vi "7.8-TCP Receive Server.vi"() -> ()   [LabVIEW 2010]
doc: "Sends a specified waveform through a TCP port. The VI first listens for a connection and, once established, sends the number of bytes to be sent followed by the data. After the data is sent, the VI waits for an 'all received' signal from the client and then breaks the connection.\n\n<B>Note:</B> Requires the Data Client.vi located in the same library as this VI."
uses:
  4-High Neurons/4.0-Timing Badass.ctl
  5-Forebrain/5.0-Global.vi
panel:
  out "Variant Cast":T1
  out "GUI":T1
  in  "Port":u16=53483 min=1025 step=1
  # "Instructions:\n1. Open the Data Client.vi\n2. Run This VI first.\n3. Run the Data Client.vi Second.\n4. Adjust the # of Points Function, and Noise Level controls.\n5. Observe the Chart on the Data Client.vi.\n6. Stop This VI. The Data Client.vi will time out and stop."
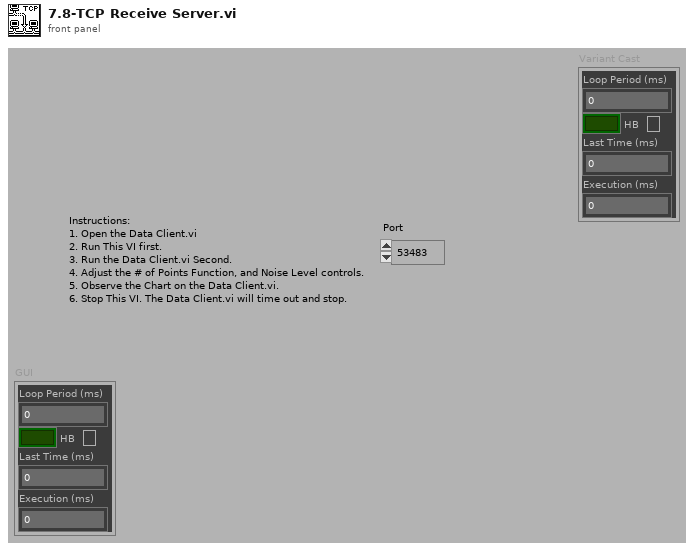
[diagram p1: front panel]
types:
  T1 = typedef "4.0-Timing Badass.ctl" = cluster{"Loop Period (ms)":u32, "HB":bool, "Last Time (ms)":u32, "Execution (ms)":u32}
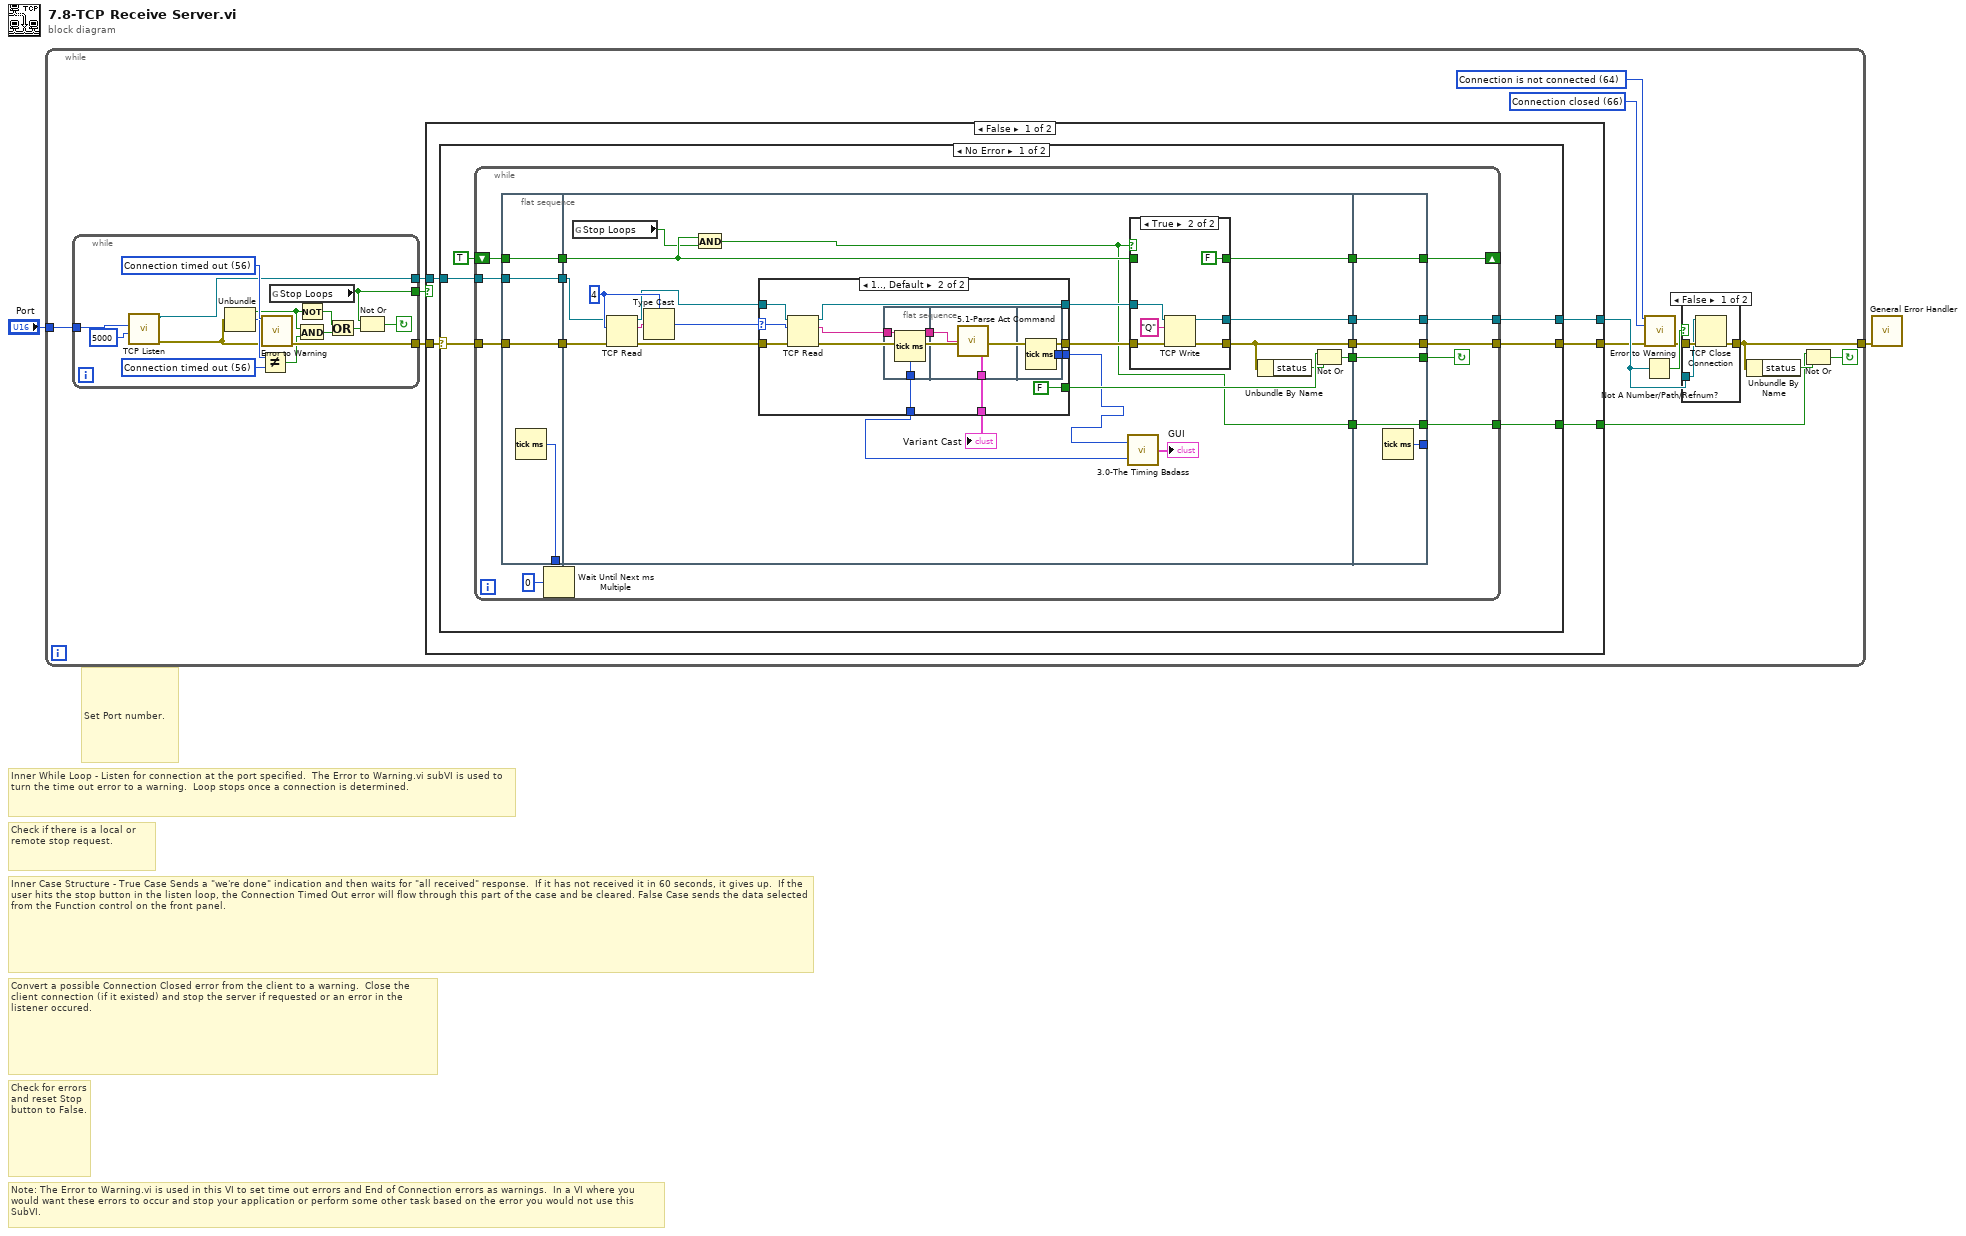
[diagram p0: block diagram]
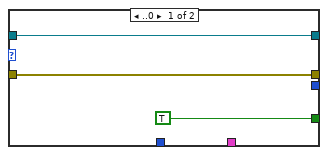
[diagram p2: hidden frame]
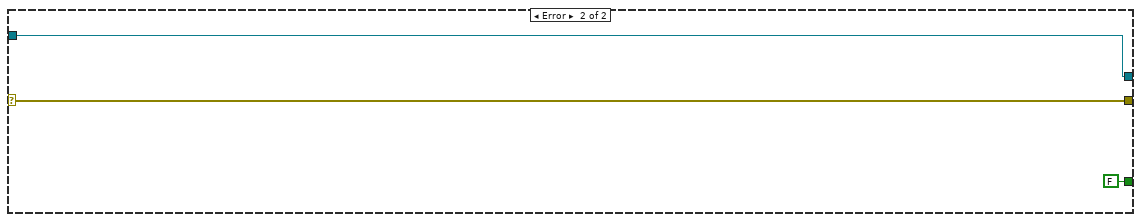
[diagram p4: hidden frame]
diagram:
  # "Check for errors\nand reset Stop \nbutton to False."
  # "Inner Case Structure - True Case Sends a \"we're done\" indication and then waits for \"all received\" response.  If it has not received it in 60 seconds, it gives up.  If the user hits the stop button in the listen loop, the Connection Timed Out error will flow through this part of the case and be cleared. False Case sends the data selected from the Function control on the front panel."
  # "Check if there is a local or remote stop request."
  # "Set Port number."
  # "Inner While Loop - Listen for connection at the port specified.  The Error to Warning.vi subVI is used to turn the time out error to a warning.  Loop stops once a connection is determined."
  # "Note: The Error to Warning.vi is used in this VI to set time out errors and End of Connection errors as warnings.  In a VI where you would want these errors to occur and stop your application or perform some other task based on the error you would not use this SubVI."
  # "Convert a possible Connection Closed error from the client to a warning.  Close the client connection (if it existed) and stop the server if requested or an error in the listener occured."
  n1 = while {
    tunnel: [w9] -> w1
    tunnel: "Port" -> [w15]
    stop <- w16 continue-if-true
    w5 = 66 items=["No Error", "Argument Error", "Memory Full", "Out of Zone", "End of File", "File Already Open", "Generic File IO Error", "File Not Found", "File Permission Error", "Disk Full", "Duplicate Path", "Too Many Files Open", "Not Enabled", "Resource File Not Found", "Cannot Add Resource", "Resource Not Found", "Image Not Found", "Image Memory Error", "Pen Does Not Exist", "Config Bad Type", "Config Token Not Found", "Config Parse Error", "Config Memory Error", "Bad External Code Format", "Bad External Code Offset", "External Code Not Present", "Null Window", "Destroy Window Mixup", "Null Menu", "Print Aborted", "Bad Print Record", "Print Driver Error", "Windows Error During Print", "Memory Error During Print", "Print Dialog Error", "Generic Print Error", "Invalid Device Refnum", "Device Not Found", "Device Parameter Error", "Device Unit Error", "Can't Open Device", "Device Call Aborted", "Generic Error", "Cancelled By User", "Object ID Too Low", "Object ID Too High", "Object Not In Heap", "Unknown Heap", "Bad DefProc ID", "DefProc Not In Table", "Message Out Of Range", "Null Method", "Unknown Message", "Manager Call Not Supported", "Bad address", "Connection In progress", "Connection timed out", "Connection is already in progress", "Network attribute not supported", "Network error", "Address in use", "System out of memory", "Connection aborted", "Connection refused", "Connection is not connected", "Connection is already connected", "Connection closed", "Initialize error (interapplication manager)", "Bad occurrence", "Wait on unbound occurrence handler", "Occurrence queue overflow", "Bad path", "Semaphore not signaled", "Unrecognized type (interapplication manager)"] ("2nd Error to Convert")
    w6 = 64 items=["No Error", "Argument Error", "Memory Full", "Out of Zone", "End of File", "File Already Open", "Generic File IO Error", "File Not Found", "File Permission Error", "Disk Full", "Duplicate Path", "Too Many Files Open", "Not Enabled", "Resource File Not Found", "Cannot Add Resource", "Resource Not Found", "Image Not Found", "Image Memory Error", "Pen Does Not Exist", "Config Bad Type", "Config Token Not Found", "Config Parse Error", "Config Memory Error", "Bad External Code Format", "Bad External Code Offset", "External Code Not Present", "Null Window", "Destroy Window Mixup", "Null Menu", "Print Aborted", "Bad Print Record", "Print Driver Error", "Windows Error During Print", "Memory Error During Print", "Print Dialog Error", "Generic Print Error", "Invalid Device Refnum", "Device Not Found", "Device Parameter Error", "Device Unit Error", "Can't Open Device", "Device Call Aborted", "Generic Error", "Cancelled By User", "Object ID Too Low", "Object ID Too High", "Object Not In Heap", "Unknown Heap", "Bad DefProc ID", "DefProc Not In Table", "Message Out Of Range", "Null Method", "Unknown Message", "Manager Call Not Supported", "Bad address", "Connection In progress", "Connection timed out", "Connection is already in progress", "Network attribute not supported", "Network error", "Address in use", "System out of memory", "Connection aborted", "Connection refused", "Connection is not connected", "Connection is already connected", "Connection closed", "Initialize error (interapplication manager)", "Bad occurrence", "Wait on unbound occurrence handler", "Occurrence queue overflow", "Bad path", "Semaphore not signaled", "Unrecognized type (interapplication manager)"] ("1st Error to Convert")
    n2 = while {
      tunnel: [w17] -> w12
      tunnel: [w28] -> w13
      tunnel: [w19] -> w14
      tunnel: w15 -> [w31]
      stop <- w29 continue-if-true
      w26 = 56 items=["No Error", "Argument Error", "Memory Full", "Out of Zone", "End of File", "File Already Open", "Generic File IO Error", "File Not Found", "File Permission Error", "Disk Full", "Duplicate Path", "Too Many Files Open", "Not Enabled", "Resource File Not Found", "Cannot Add Resource", "Resource Not Found", "Image Not Found", "Image Memory Error", "Pen Does Not Exist", "Config Bad Type", "Config Token Not Found", "Config Parse Error", "Config Memory Error", "Bad External Code Format", "Bad External Code Offset", "External Code Not Present", "Null Window", "Destroy Window Mixup", "Null Menu", "Print Aborted", "Bad Print Record", "Print Driver Error", "Windows Error During Print", "Memory Error During Print", "Print Dialog Error", "Generic Print Error", "Invalid Device Refnum", "Device Not Found", "Device Parameter Error", "Device Unit Error", "Can't Open Device", "Device Call Aborted", "Generic Error", "Cancelled By User", "Object ID Too Low", "Object ID Too High", "Object Not In Heap", "Unknown Heap", "Bad DefProc ID", "DefProc Not In Table", "Message Out Of Range", "Null Method", "Unknown Message", "Manager Call Not Supported", "Bad address", "Connection In progress", "Connection timed out", "Connection is already in progress", "Network attribute not supported", "Network error", "Address in use", "System out of memory", "Connection aborted", "Connection refused", "Connection is not connected", "Connection is already connected", "Connection closed", "Initialize error (interapplication manager)", "Bad occurrence", "Wait on unbound occurrence handler", "Occurrence queue overflow", "Bad path", "Semaphore not signaled", "Unrecognized type (interapplication manager)"] ("1st Error to Convert")
      w27 = 56 items=["No Error", "Argument Error", "Memory Full", "Out of Zone", "End of File", "File Already Open", "Generic File IO Error", "File Not Found", "File Permission Error", "Disk Full", "Duplicate Path", "Too Many Files Open", "Not Enabled", "Resource File Not Found", "Cannot Add Resource", "Resource Not Found", "Image Not Found", "Image Memory Error", "Pen Does Not Exist", "Config Bad Type", "Config Token Not Found", "Config Parse Error", "Config Memory Error", "Bad External Code Format", "Bad External Code Offset", "External Code Not Present", "Null Window", "Destroy Window Mixup", "Null Menu", "Print Aborted", "Bad Print Record", "Print Driver Error", "Windows Error During Print", "Memory Error During Print", "Print Dialog Error", "Generic Print Error", "Invalid Device Refnum", "Device Not Found", "Device Parameter Error", "Device Unit Error", "Can't Open Device", "Device Call Aborted", "Generic Error", "Cancelled By User", "Object ID Too Low", "Object ID Too High", "Object Not In Heap", "Unknown Heap", "Bad DefProc ID", "DefProc Not In Table", "Message Out Of Range", "Null Method", "Unknown Message", "Manager Call Not Supported", "Bad address", "Connection In progress", "Connection timed out", "Connection is already in progress", "Network attribute not supported", "Network error", "Address in use", "System out of memory", "Connection aborted", "Connection refused", "Connection is not connected", "Connection is already connected", "Connection closed", "Initialize error (interapplication manager)", "Bad occurrence", "Wait on unbound occurrence handler", "Occurrence queue overflow", "Bad path", "Semaphore not signaled", "Unrecognized type (interapplication manager)"] ("1st Error to Convert")
      n3 = call <vilib>:"TCP Listen.vi"("timeout ms (wait forever: -1)"=5000, "port"=w31) -> ("error out"=w18:errorcluster, "connection ID"=w19:refnum<k5>)  [unwired: 6 in, 2 out]
      n4 = Unbundle(w18) -> ("status"=w24:bool, "code"=w25:i32)  [unwired: 1 out]
      n5 = Not Equal?(x=w25, y=w26) -> (x != y?=w23:bool)
      n6 = call <vilib>:"Error to Warning.vi"("1st Error to Convert"=w27, "error in"=w18) -> ("warning out"=w28:errorcluster)  [unwired: 13 in]
      n7 = global read "5.0-Global.vi" "Stop Loops"() -> (w17:bool)
      n8 = Not(x=w24) -> (.not. x?=w22:bool)
      n9 = And(x=w24, y=w23) -> (x .and. y?=w21:bool)
      n10 = Or(x=w22, y=w21) -> (x .or. y?=w20:bool)
      n11 = Not Or(1:w20, 2:w17) -> (0:w29:bool)
    }
    n12 = case shown="False" w12 {
      selector: w12 -> [_ w123]
      tunnel: [w36 w124] -> w4
      tunnel: w14 -> [w35 w125]
      tunnel: w13 -> [w32 w124]
      tunnel: [w34 w125] -> w11
      tunnel: [w33 w123] -> w7
      frame False {
        n13 = case shown="No Error" w32 {
          selector: w32 -> [w41 w120]
          tunnel: [w39 w120] -> w36
          tunnel: w35 -> [w42 w122]
          tunnel: [w40 w122] -> w34
          tunnel: [w38 FALSE] -> w33
          frame No Error {
            n14 = while {
              shift-left: TRUE -> [w56]
              shift-right: [w58] -> _
              tunnel: [w57] -> w40
              tunnel: [w55] -> w39
              tunnel: w42 -> [w54]
              tunnel: w41 -> [w53]
              tunnel: [w52] -> w38
              stop <- w59 continue-if-true
              n15 = flat-sequence {
                tunnel: w53 -> [w61]
                tunnel: w54 -> [w62]
                tunnel: w56 -> [w63]
                tunnel: [w63] -> w46
                tunnel: [w62] -> w45
                tunnel: [w61] -> w44
                tunnel: [w60] -> _
                tunnel: [w84] -> w51
                tunnel: [w81] -> w50
                tunnel: [w76] -> w49
                tunnel: [w73] -> w48
                tunnel: [w64] -> w47
                tunnel: w46 -> [w74]
                tunnel: w45 -> [w71]
                tunnel: w44 -> [w70]
                tunnel: [w115] -> w52
                tunnel: [w116] -> w55
                tunnel: [w117] -> w57
                tunnel: [w118] -> w58
                tunnel: [w119] -> w59
                tunnel: w51 -> [w119]
                tunnel: w50 -> [w118]
                tunnel: w49 -> [w117]
                tunnel: w48 -> [w116]
                tunnel: w47 -> [w115]
                tunnel: [w114] -> _
                frame #0 {
                  n16 = Tick Count (ms)() -> (millisecond timer value=w60:u32)
                }
                frame #1 {
                  w83 = 4
                  n17 = global read "5.0-Global.vi" "Stop Loops"() -> (w65:bool)
                  n18 = TCP Read(connection ID=w71, bytes to read=w83, error in (no error)=w70) -> (connection ID out=w77:refnum<k5>, data out=w85:string, error out=w78:errorcluster)  [unwired: 2 out]
                  n19 = Type Cast(type=w83, x=w85) -> (*(type *) &x=w82:i32)
                  n20 = And(x=w74, y=w65) -> (x .and. y?=w64:bool)
                  n21 = case shown="1.., Default" w82 {
                    selector: w82 -> [_ w96]
                    tunnel: w78 -> [w86 w99]
                    tunnel: w77 -> [w88 w98]
                    tunnel: [w88 w97] -> w75
                    tunnel: [TRUE FALSE] -> w79
                    tunnel: [w86 w94] -> w80
                    tunnel: [_ w91] -> w68
                    tunnel: [_ w90] -> w67
                    tunnel: [_ w89] -> w66
                    frame ..0 {
                    }
                    frame 1.., Default {
                      n22 = TCP Read(connection ID=w98, bytes to read=w96, error in (no error)=w99) -> (connection ID out=w97:refnum<k5>, data out=w93:string, error out=w94:errorcluster)  [unwired: 2 out]
                      n23 = flat-sequence {
                        tunnel: w93 -> [w101]
                        tunnel: [w101] -> w92
                        tunnel: [w100] -> w90
                        tunnel: w92 -> [w103]
                        tunnel: [w102] -> w89
                        tunnel: [w104] -> w91
                        frame #0 {
                          n24 = Tick Count (ms)() -> (millisecond timer value=w100:u32)
                        }
                        frame #1 {
                          n25 = call "5.1-Parse Act Command.vi"("data out"=w103) -> ("GUI"=w102:T1)
                        }
                        frame #2 {
                          n26 = Tick Count (ms)() -> (millisecond timer value=w104:u32)
                        }
                      }
                    }
                  }
                  "Variant Cast" <- w66
                  n27 = call "3.0-The Timing Badass.vi"("Start"=w67, "End"=w68) -> ("Super Heart Beat"=→"GUI":T1)
                  n28 = case shown="True" w64 {
                    tunnel: w74 -> [w106 _]
                    tunnel: [w106 FALSE] -> w81
                    tunnel: w75 -> [w105 w113]
                    tunnel: w80 -> [w107 w110]
                    tunnel: [w107 w109] -> w73
                    tunnel: [w105 w108] -> w76
                    frame False {
                    }
                    frame True {
                      n29 = TCP Write(connection ID=w113, data in="Q", error in (no error)=w110) -> (connection ID out=w108:refnum<k5>, error out=w109:errorcluster)  [unwired: 2 out]
                    }
                  }
                  n30 = Unbundle By Name(w73) -> ("status"=w72:bool)
                  n31 = Not Or(1:w72, 2:w79) -> (0:w84:bool)
                }
                frame #2 {
                  n32 = Tick Count (ms)() -> (millisecond timer value=w114:u32)
                }
              }
              n33 = Wait Until Next ms Multiple(millisecond multiple=u32 0) -> ()  [unwired: 1 out]
            }
          }
          frame Error {
          }
        }
      }
      frame True {
      }
    }
    n34 = Not A Number/Path/Refnum?(number/path/refnum=w11) -> (NaN/Path/Refnum?=w10:bool)
    n35 = call <vilib>:"Error to Warning.vi"("1st Error to Convert"=w6, "2nd Error to Convert"=w5, "error in"=w4) -> ("warning out"=w3:errorcluster)  [unwired: 12 in]
    n36 = case shown="False" w10 {
      tunnel: w3 -> [w128 w129]
      tunnel: w11 -> [w127 _]
      tunnel: [w126 w129] -> w9
      frame False {
        n37 = TCP Close Connection(connection ID=w127, error in (no error)=w128) -> (error out=w126:errorcluster)  [unwired: 1 in, 1 out]
      }
      frame True {
      }
    }
    n38 = Unbundle By Name(w9) -> ("status"=w8:bool)
    n39 = Not Or(1:w8, 2:w7) -> (0:w16:bool)
  }
  n40 = call <vilib>:"General Error Handler.vi"("error in (no error)"=w1) -> ()  [unwired: 10 in, 5 out]
